vi "schednamecreator.vi"   [LabVIEW 2023]
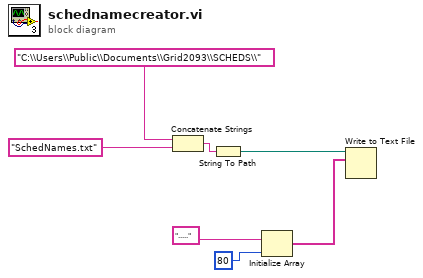
[diagram p0: block diagram]
diagram:
  n1 = Concatenate Strings("C:\\Users\\Public\\Documents\\Grid2093\\SCHEDS\\", "SchedNames.txt" ("string")) -> (w6:string)
  n2 = String To Path(string=w6) -> (path=w7:path)
  n3 = Initialize Array(".....", 80 ("y")) -> (w1:string[])
  n4 = Write to Text File(file (use dialog)=w7, text=w1) -> ()  [unwired: 2 in, 3 out]
